vi "Query Stop Notifier.vi"(10 "Time Out":i32, 11 "System Actor in":refnum<class "System Actor.lvclass">) -> (1 "Time Out?":bool, 2 "notification":i64, 3 "System Actor out":refnum<class "System Actor.lvclass">)   [LabVIEW 2024, in "System Actor.lvclass"]
uses:
  System Actor.lvclass
  System Actor.lvclass/System Actor.ctl
  Actor Assistant/Notifier/Convert Notification/Instance/I64.vi
  Actor Assistant/Notifier/Notifier.lvclass
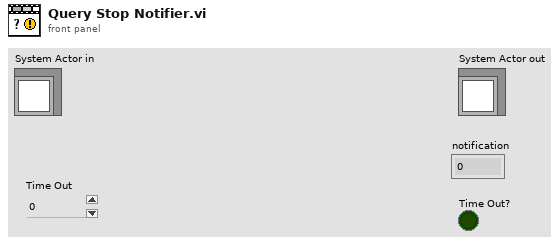
[diagram p1: front panel]
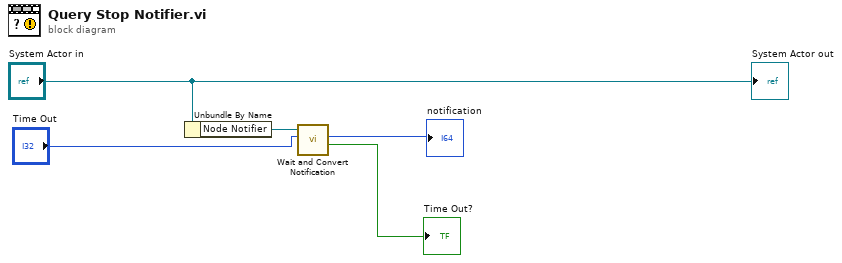
[diagram p0: block diagram]
diagram:
  n1 = Unbundle By Name("System Actor in") -> ("Node Notifier"=w4:refnum<class "Notifier.lvclass">)
  n2 = call-poly "Wait and Convert Notification.vi"("Timeout"="Time Out", "Notifier in"=w4) -> ("Timeout?"=→"Time Out?":bool, "Notification Out"=→"notification":i64)  [unwired: 6 in, 2 out]
  "System Actor out" <- "System Actor in"
